vi "HTML Report.vi"() -> ()   [LabVIEW 2020]
doc: "This is an example of some of the new things that you can do with HTML reports. \nIt adds objects other than just normal text to a report. For an example of the text capabilities of LabVIEW's report generation VIs, you should look at the Text Report Example."
uses:
  <vilib>/Utility/NIReport.llb/NI_report.lvclass
  <vilib>/Utility/NIReport.llb/HTML Report Image Alignment.ctl
  <vilib>/Utility/NIReport.llb/NI_ReportGenerationCore.lvlib
  <vilib>/Utility/NIReport.llb/Append Report Text (str wrap).vi
  <vilib>/printing/ReportDocExtensions.llb/Append Front Panel Image to Report (path).vi
  <vilib>/printing/OpenHTMLReport.llb/Open HTML Report in Browser (Path).vi
panel:
  in  "String":string="<tab>This is an example of some of the new things that you can do with HTML reports.  It concentrates on things other than just normal text.  For an example of the text capabilities of LabVIEW's report generation VIs, you should look at the Text Report Example. <newline> <tab>Above is a copy of the Waveform Chart Control from Strip Chart.vi.  Below is a horizontal line.  Below the line is the front panel of Strip Chart.vi.  Next to that is a link to NI's homepage.  And finally, there is a piece of Java Script inserted to give the date when the page was saved.<newline>"
  in  "HTML Save Path":path caption="HTML Save Path (if empty, uses example.html in temp directory)"
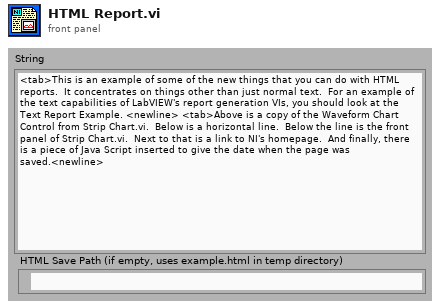
[diagram p1: front panel]
types:
  T1 = typedef "NI_ReportGenerationCore.lvlib/HTML Report Image Alignment.ctl" = enum16{"(default)", "LEFT", "RIGHT", "TOP", "TEXTTOP", "MIDDLE", "ABSMIDDLE", "BASELINE", "BOTTOM", "ABSBOTTOM"}
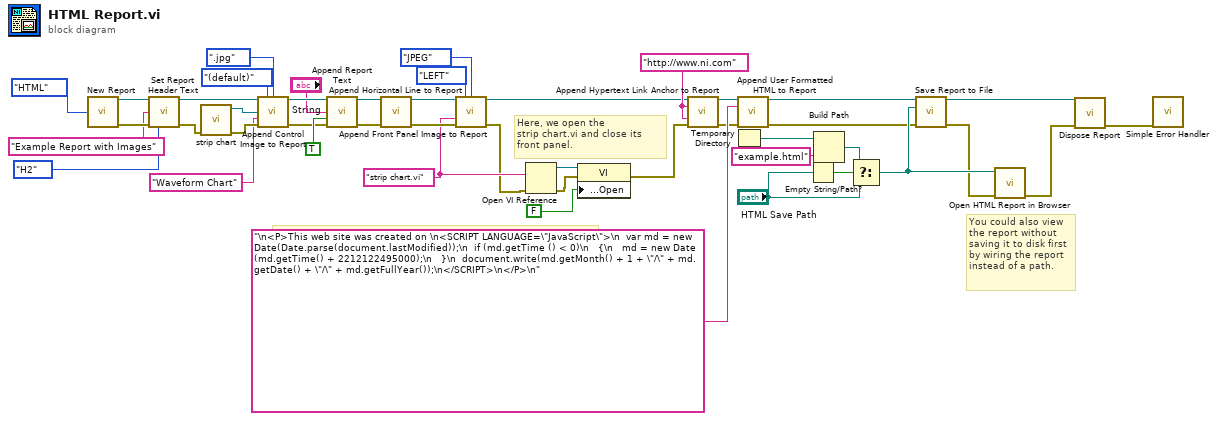
[diagram p0: block diagram]
diagram:
  w9 = "strip chart.vi"
  w43 = "http://www.ni.com" ("URL of link - href")
  # "Here, we open the \nstrip chart.vi and close its\nfront panel."
  # "You could also view\nthe report without\nsaving it to disk first\nby wiring the report\ninstead of a path."
  # "Java Script inserted to give the date when the page was saved"
  n1 = call <vilib>:"New Report.vi"("report type"=enum16{"Standard Report", "HTML"}."HTML") -> ("report out"=w33:refnum<class "NI_report.lvclass">, "error out"=w34:errorcluster)  [unwired: 13 in]
  n2 = call-dynamic "Set Report Header Text.vi"("report in"=w33, "center header text"="Example Report with Images", "error in (no error)"=w34, "HTML header size"=enum16{"H1", "H2", "H3", "H4", "H5", "H6", "H7"}."H2") -> ("report out"=w17:refnum<class "NI_report.lvclass">, "error out"=w16:errorcluster)  [unwired: 10 in]
  n3 = call "strip chart.vi"("error in (no error)"=w16) -> ("error out"=w25:errorcluster, "Ctrl Reference"=w15:refnum<vi>)  [unwired: 4 in, 1 out]
  n4 = call-dynamic "Append Control Image to Report.vi"("report in"=w17, "alignment (default)"=HTML_Report_Image_Alignment."(default)", "image file type (.jpg)"=enum16{".jpg", ".png"}.".jpg" ("image file type"), "ctrl reference"=w15, "description"="Waveform Chart" ("control name"), "error in (no error)"=w25) -> ("report out"=w24:refnum<class "NI_report.lvclass">, "error out"=w26:errorcluster)  [unwired: 6 in, 2 out]
  n5 = call-poly <vilib>:"Append Report Text.vi"("report in"=w24, "text"="String", "append on new line? (F)"=TRUE, "error in (no error)"=w26) -> ("report out"=w21:refnum<class "NI_report.lvclass">, "error out"=w20:errorcluster)  [unwired: 8 in, 2 out]
  n6 = call-dynamic "Append Horizontal Line to Report.vi"("report in"=w21, "error in (no error)"=w20) -> ("report out"=w18:refnum<class "NI_report.lvclass">, "error out"=w19:errorcluster)  [unwired: 12 in]
  n7 = call-poly <vilib>:"Append Front Panel Image to Report.vi"("report in"=w18, "alignment (default)"=HTML_Report_Image_Alignment."LEFT", "image format (jpeg)"=enum32{"PNG", "JPEG", "GIF"}."JPEG" ("Image Format (jpeg)"), "description"=w9, "error in (no error)"=w19) -> ("report out"=w10:refnum<class "NI_report.lvclass">, "error out"=w8:errorcluster)  [unwired: 6 in, 3 out]
  n8 = Open VI Reference(vi path=w9, error in (no error)=w8) -> (vi reference=w7:refnum<vi>, error out=w6:errorcluster)  [unwired: 4 in]
  n9 = property class="VI"(reference=w7, error in=w6, "Front Panel Window:Open"=FALSE) -> (error out=w4:errorcluster)  [unwired: 1 out]
  n10 = call-dynamic "Append Hypertext Link Anchor to Report.vi"("report in"=w10, "URL of link - href"=w43, "link text"=w43, "error in (no error)"=w4) -> ("report out"=w23:refnum<class "NI_report.lvclass">, "error out"=w22:errorcluster)  [unwired: 8 in, 2 out]
  n11 = Temporary Directory() -> (w41:path)
  n12 = call-dynamic "Append User Formatted HTML to Report.vi"("report in"=w23, "HTML text"="\n<P>This web site was created on \n<SCRIPT LANGUAGE=\"JavaScript\">\n  var md = new Date(Date.parse(document.lastModified));\n  if (md.getTime () < 0)\n   {\n   md = new Date (md.getTime() + 2212122495000);\n   }\n  document.write(md.getMonth() + 1 + \"/\" + md.getDate() + \"/\" + md.getFullYear());\n</SCRIPT>\n</P>\n", "error in (no error)"=w22) -> ("report out"=w13:refnum<class "NI_report.lvclass">, "error out"=w12:errorcluster)  [unwired: 11 in]
  n13 = Empty String/Path?(string/path="HTML Save Path") -> (empty?=w39:bool)
  n14 = Build Path(base path=w41, name or relative path="example.html") -> (appended path=w38:path)
  n15 = Select(t=w38, s=w39, f="HTML Save Path") -> (s? t:f=w36:path)
  n16 = call-dynamic "Save Report to File.vi"("report in"=w13, "report file path"=w36, "error in (no error)"=w12) -> ("report out"=w44:refnum<class "NI_report.lvclass">, "error out"=w14:errorcluster)  [unwired: 11 in]
  n17 = call-poly <vilib>:"Open HTML Report in Browser.vi"("path"=w36, "error in (no error)"=w14) -> ("error out"=w45:errorcluster)  [unwired: 12 in, 1 out]
  n18 = call-dynamic "Dispose Report.vi"("report in"=w44, "error in (no error)"=w45) -> ("error out"=w3:errorcluster)  [unwired: 13 in]
  n19 = call <vilib>:"Simple Error Handler.vi"("error in (no error)"=w3) -> ()  [unwired: 4 in, 5 out]
